vi "ON-OFF Cycle Control (SubVI).vi"(0 "ON Time (s)":dbl=10.0, 1 "OFF Time (s)":dbl=10.0, 2 "Cycle Limit":i32=100, 5 "Reset Cycle Count":bool) -> (14 "State Output (ON / OFF)":bool, 15 "Elapsed State Time (s)":dbl format="%.1f", 16 "Total Elapsed Time (s)":dbl format="%.1f", 17 "Cycle Count":i32, 18 "Time Remaining (s)":dbl format="%.1f")   [LabVIEW 2009]
panel:
  # "ON-OFF Cycle Control (SubVI)\nCreated by Blake Otting\n4/15/2010"
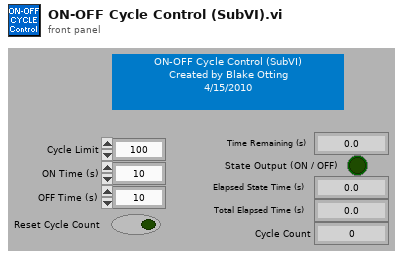
[diagram p1: front panel]
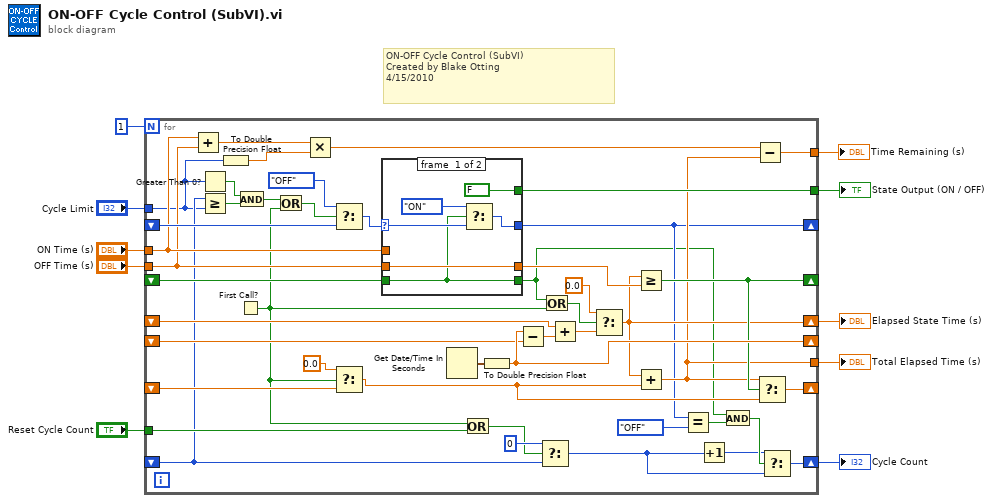
[diagram p0: block diagram]
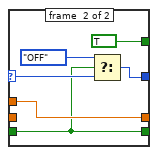
[diagram p2: hidden frame]
diagram:
  # "ON-OFF Cycle Control (SubVI)\nCreated by Blake Otting\n4/15/2010"
  n1 = for {
    N: 1 -> [_]
    shift-right: [w34] -> _
    shift-left: _ -> [w55]
    shift-right: [w14] -> _
    shift-left: _ -> [w51]
    tunnel: "ON Time (s)" -> [w29]
    tunnel: "OFF Time (s)" -> [w28]
    tunnel: [w53] -> w2
    shift-right: [w45] -> w7
    shift-left: _ -> [w27]
    tunnel: "Reset Cycle Count" -> [w43]
    shift-right: [w33] -> w8
    shift-left: _ -> [w41]
    shift-right: [w40] -> _
    shift-left: _ -> [w39]
    shift-right: [w21] -> _
    shift-left: _ -> [w30]
    tunnel: "Cycle Limit" -> [w19]
    tunnel: [w20] -> w10
    tunnel: [w15] -> w1
    n2 = Add(x=w29, y=w28) -> (x+y=w24:dbl)
    n3 = Greater Than 0?(x=w19) -> (x > 0?=w18:bool)
    n4 = Greater Or Equal?(x=w27, y=w19) -> (x >= y?=w17:bool)
    n5 = To Double Precision Float(number=w19) -> (double precision float=w23:dbl)
    n6 = First Call?() -> (First Call?: T/F=w26:bool)
    n7 = And(x=w18, y=w17) -> (x .and. y?=w16:bool)
    n8 = Or(x=w16, y=w26) -> (x .or. y?=w25:bool)
    n9 = Multiply(x=w24, y=w23) -> (x*y=w22:dbl)
    n10 = Select(t=enum16{"OFF", "ON"}."OFF" ("Mode (Read)"), s=w25, f=w51) -> (s? t:f=w13:enum16{"OFF", "ON"})
    n11 = Select(t=0.0, s=w26, f=w30) -> (s? t:f=w31:dbl)
    n12 = case shown="\"OFF\", Default" w13 {
      selector: w13 -> [w59 w65]
      tunnel: w55 -> [w57 w63]
      tunnel: [w60 w66] -> w14
      tunnel: w29 -> [_ w64]
      tunnel: [w58 w64] -> w54
      tunnel: w28 -> [w58 _]
      tunnel: [w57 w63] -> w11
      tunnel: [FALSE TRUE] -> w53
      frame #0 {
        n13 = Select(t=enum16{"OFF", "ON"}."ON" ("Mode (Read)"), s=w57, f=w59) -> (s? t:f=w60:enum16{"OFF", "ON"})
      }
      frame #1 {
        n14 = Select(t=enum16{"OFF", "ON"}."OFF" ("Mode (Read)"), s=w63, f=w65) -> (s? t:f=w66:enum16{"OFF", "ON"})
      }
    }
    n15 = Get Date/Time In Seconds() -> (seconds since 1Jan1904=w38:timestamp)
    n16 = Or(x=w26, y=w43) -> (x .or. y?=w42:bool)
    n17 = To Double Precision Float(number=w38) -> (double precision float=w40:dbl)
    n18 = Subtract(x=w40, y=w39) -> (x-y=w37:dbl)
    n19 = Select(t=0, s=w42, f=w27) -> (s? t:f=w46:i32)
    n20 = Or(x=w11, y=w26) -> (x .or. y?=w12:bool)
    n21 = Add(x=w41, y=w37) -> (x+y=w36:dbl)
    n22 = Select(t=0.0, s=w12, f=w36) -> (s? t:f=w33:dbl)
    n23 = Greater Or Equal?(x=w33, y=w54) -> (x >= y?=w34:bool)
    n24 = Add(x=w33, y=w31) -> (x+y=w15:dbl)
    n25 = Equal?(x=w14, y=enum16{"OFF", "ON"}."OFF") -> (x = y?=w49:bool)
    n26 = Increment(x=w46) -> (x+1=w44:i32)
    n27 = And(x=w11, y=w49) -> (x .and. y?=w48:bool)
    n28 = Subtract(x=w22, y=w15) -> (x-y=w20:dbl)
    n29 = Select(t=w15, s=w34, f=w31) -> (s? t:f=w21:dbl)
    n30 = Select(t=w44, s=w48, f=w46) -> (s? t:f=w45:i32)
  }
  "Elapsed State Time (s)" <- w8
  "State Output (ON / OFF)" <- w2
  "Cycle Count" <- w7
  "Total Elapsed Time (s)" <- w1
  "Time Remaining (s)" <- w10
